vi "q4 compound interest.vi"() -> ()   [LabVIEW 2025]
panel:
  out "CI":dbl
  in  "FORMULA":string
  in  "T":dbl
  in  "R":dbl
  in  "P":dbl
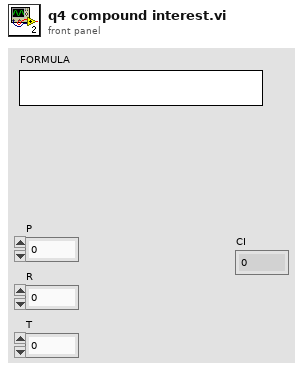
[diagram p1: front panel]
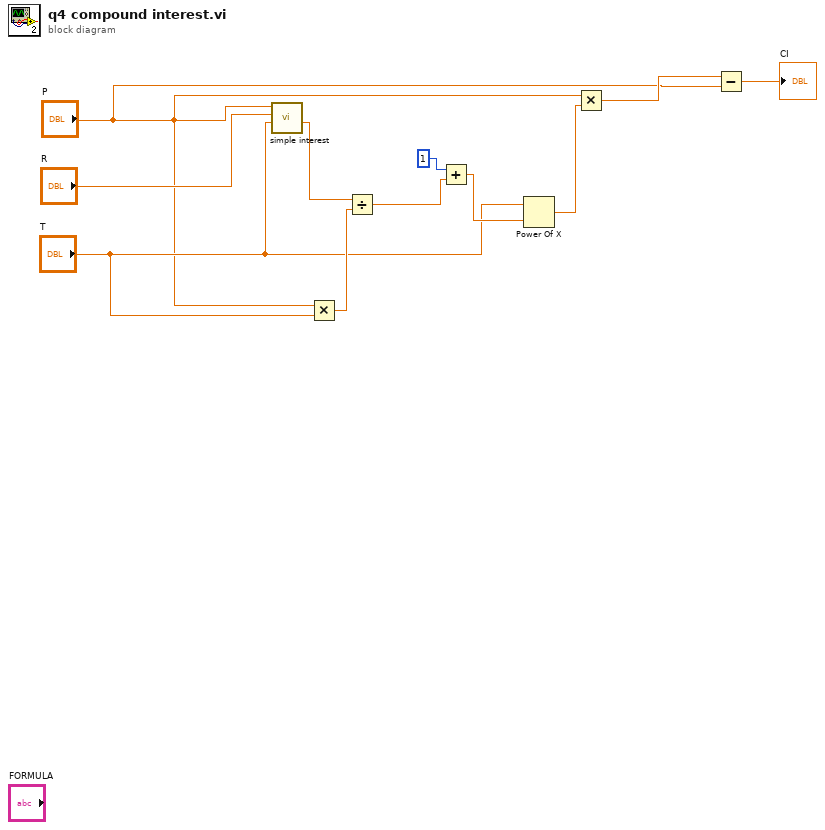
[diagram p0: block diagram]
diagram:
  n1 = call "simple interest.vi"("T"="T", "R"="R", "P"="P") -> ("SI"=w10:dbl)  [unwired: 8 in]
  n2 = Multiply(x="P", y="T") -> (x*y=w9:dbl)
  n3 = Divide(x=w10, y=w9) -> (x/y=w8:dbl)
  n4 = Add(x=1, y=w8) -> (x+y=w6:dbl)
  n5 = Power Of X(1:w6, 2:"T") -> (0:w4:dbl)
  n6 = Multiply(x="P", y=w4) -> (x*y=w3:dbl)
  n7 = Subtract(x=w3, y="P") -> (x-y=→"CI":dbl)
